vi "Begin.vi"(11 "Image Size":T1=enum."160x120") -> (0 "error out":errorcluster)   [LabVIEW 2012]
doc: "Called before other user functions, this VI is expected to open initial I/O refnums, load in file data, and do all program initialization. Notice that the <B>error out</B> terminal is simply used for data flow. Wiring it to other structures or subVIs ensures that this VI runs first."
uses:
  <vilib>/Rock Robotics/WPI/Camera/WPI_CameraImageSize.ctl
  <vilib>/Rock Robotics/WPI/DriverStation/WPI_DriverStationRobotMode2.ctl
  <vilib>/Rock Robotics/WPI/CAN/Jaguar/SubVIs/WPI_CANJaguar_ControlMode.ctl
  <vilib>/Rock Robotics/WPI/Joystick/WPI_JoystickDeviceEnum.ctl
  <vilib>/Rock Robotics/WPI/CAN/Jaguar/SubVIs/WPI_CANJaguar_SpeedReference.ctl
  Robot Global Data.vi
  <vilib>/Rock Robotics/WPI/MotorControl/WPI_MotorControlOpenCANJaguar.vi
  <vilib>/Rock Robotics/WPI/RobotDrive/WPI_RobotDriveOpen2MotorWithJaguar.vi
  <vilib>/Rock Robotics/SystemInterfaces/DIO/FPGA_DIOPWMChannel.ctl
  <vilib>/Rock Robotics/WPI/Camera/WPI_CameraWhite Balance Values.ctl
  <vilib>/Rock Robotics/WPI/Camera/WPI_CameraExposure Values.ctl
  <vilib>/Rock Robotics/WPI/Camera/WPI_CameraFrameRate.ctl
  <vilib>/Rock Robotics/WPI/SafetyOutput/WPI_SafetyOutputConfigMenu.ctl
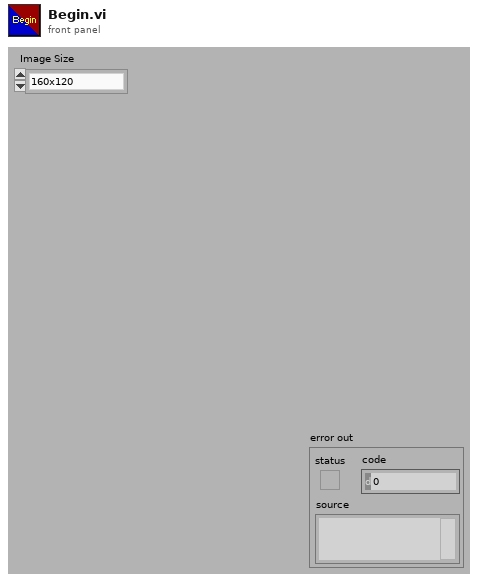
[diagram p1: front panel]
types:
  T1 = typedef "WPI_CameraImageSize.ctl" = enum16{"640x480", "320x240", "160x120"}
  T2 = typedef "WPI_CANJaguar_SpeedReference.ctl" = u8
  T3 = typedef "WPI_CANJaguar_ControlMode.ctl" = enum8{"Percent VBus", "Current", "Speed", "Position", "Voltage"}
  T4 = typedef "WPI_JoystickDeviceEnum.ctl" = enum16{"USB 1", "USB 2", "USB 3", "USB 4", "Kinect 1", "Kinect 2"}
  T5 = typedef "WPI_DriverStationRobotMode2.ctl" = enum16{"Autonomous Disabled", "Autonomous Enabled", "Teleop Disabled", "Teleop Enabled", "Timeout", "Finish", "Test Disabled", "Test Enabled"}
  T6 = typedef "WPI_CameraFrameRate.ctl" = u32
  T7 = typedef "WPI_CameraExposure Values.ctl" = enum16{"Auto", "Flicker-free 50 Hz", "Flicker-free 60 Hz", "Hold current"}
  T8 = typedef "WPI_CameraWhite Balance Values.ctl" = enum16{"Auto", "Fixed indoor", "Fixed outdoor 1", "Fixed outdoor 2", "Fixed fluorescent 1", "Fixed fluorescent 2", "Hold current"}
  T9 = typedef "WPI_CameraDevRef.ctl" = cluster{"Camera Address":string, "CameraStatus":errorcluster, "Acquire Image Notifier":refnum<notifier>}
  T10 = typedef "WPI_SafetyOutputConfigMenu.ctl" = enum16{"Enable", "Disable"}
  T11 = typedef "FPGA_DIOPWMChannel.ctl" = enum8{"PWM 1", "PWM 2", "PWM 3", "PWM 4", "PWM 5", "PWM 6", "PWM 7", "PWM 8", "PWM 9", "PWM 10", "Invalid"}
  T12 = typedef "WPI_JoystickDevRef.ctl" = cluster{"Device":T4}
  T13 = typedef "WPI_RobotDriveDevRef.ctl" = cluster{"DevStatus":errorcluster, "Motors[]":T14[], "Square Inputs":bool, "Max Output":dbl, "Isochronous":bool}
  T14 = typedef "WPI_MotorControlDeviceRef.ctl" = cluster{"DeviceStatus":errorcluster, "Type":enum16{"PWM", "CAN"}, "PWM":cluster{"Digital Module":T15, "PWM Channel":T11, "DeadBand":T16}, "CAN":cluster{"Device Number":u8, "Control Mode":T3, "Semaphore":T17, "Max Vout":dbl}, "Invert":bool, "TransformRef":T18, "InvTransformRef":T18}
  T15 = typedef "FPGA_TypedefDigitalModule.ctl" = enum16{"Digital Module 1", "Digital Module 2"}
  T16 = typedef "WPI_PWMDeadband.ctl" = cluster{"Name":string, "maxPositivePwm":i32, "minPositivePwm":i32, "centerPwm":i32, "maxNegativePwm":i32, "minNegativePwm":i32, "angularRange":u16}
  T17 = typedef "Semaphore RefNum" = refnum<k1>
  T18 = typedef "WPI_PWMTransform_ConPane.ctl" = refnum<vi>
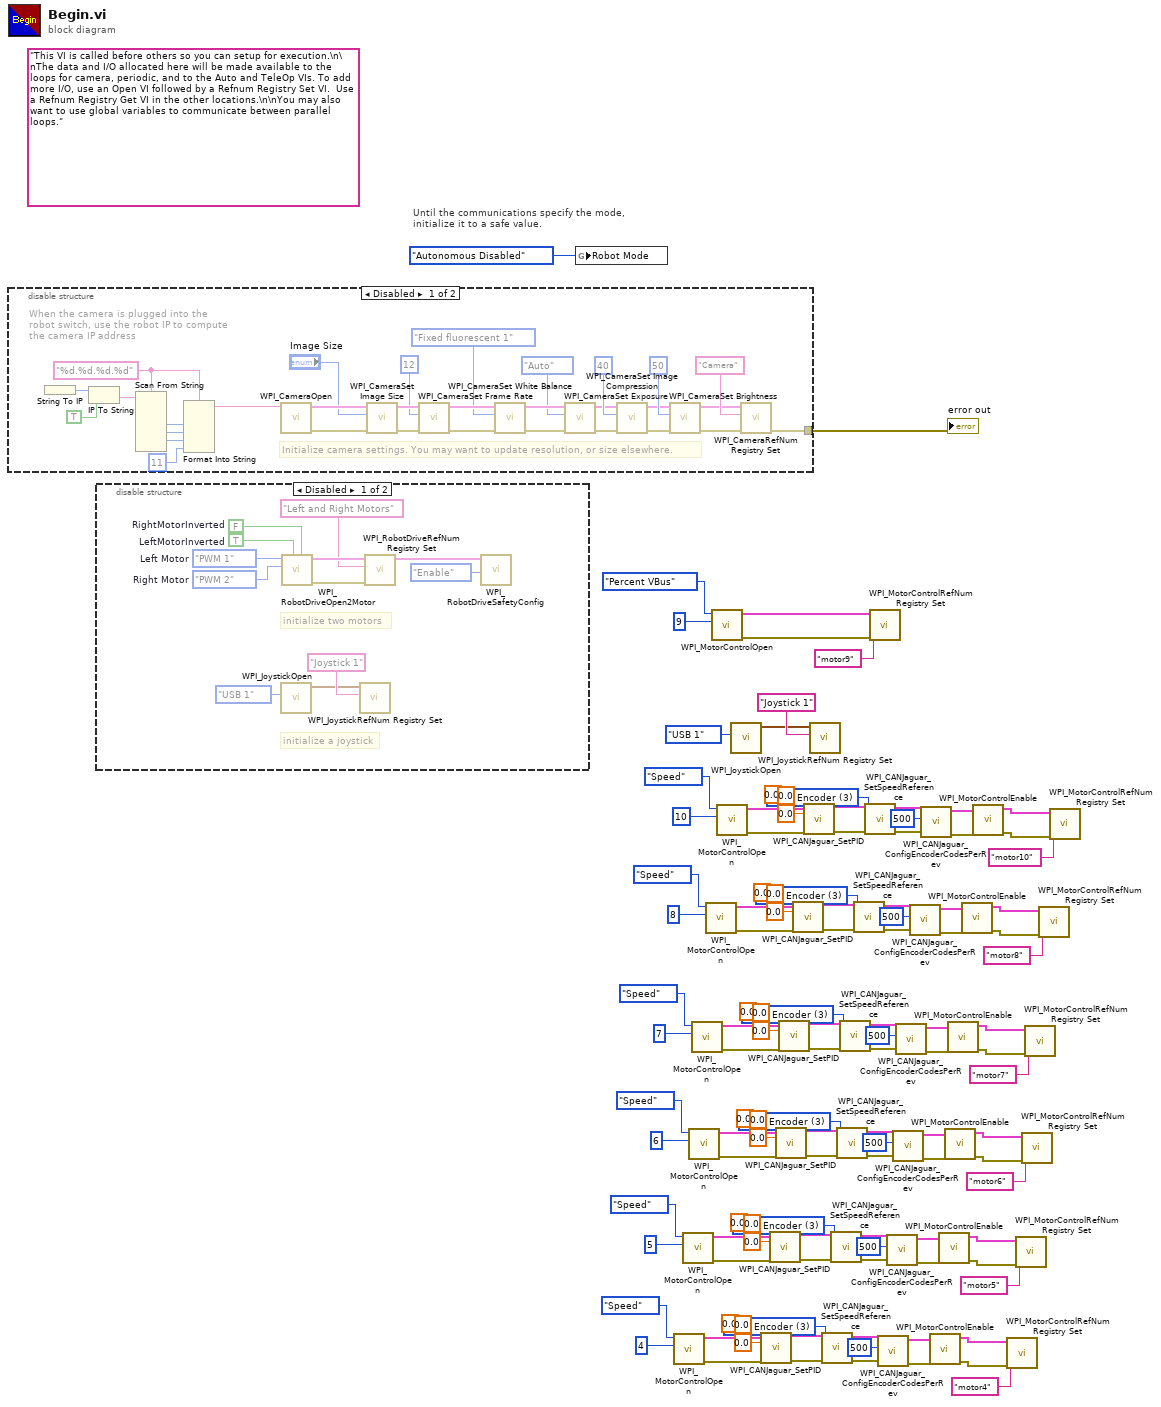
[diagram p0: block diagram]
diagram:
  w9 = T2 3 items=["Encoder"=0, "Inv Encoder"=2, "Quad Encoder"=3, "None"=255] ("Speed Reference")
  w27 = T2 3 items=["Encoder"=0, "Inv Encoder"=2, "Quad Encoder"=3, "None"=255] ("Speed Reference")
  w45 = T2 3 items=["Encoder"=0, "Inv Encoder"=2, "Quad Encoder"=3, "None"=255] ("Speed Reference")
  w63 = T2 3 items=["Encoder"=0, "Inv Encoder"=2, "Quad Encoder"=3, "None"=255] ("Speed Reference")
  w81 = T2 3 items=["Encoder"=0, "Inv Encoder"=2, "Quad Encoder"=3, "None"=255] ("Speed Reference")
  w99 = T2 3 items=["Encoder"=0, "Inv Encoder"=2, "Quad Encoder"=3, "None"=255] ("Speed Reference")
  (unwired) "This VI is called before others so you can setup for execution.\n\nThe data and I/O allocated here will be made available to the loops for camera, periodic, and to the Auto and TeleOp VIs. To add more I/O, use an Open VI followed by a Refnum Registry Set VI.  Use a Refnum Registry Get VI in the other locations.\n\nYou may also want to use global variables to communicate between parallel loops."
  # "Until the communications specify the mode,\ninitialize it to a safe value."
  n1 = disable-structure shown="Disabled" {
    disable-tunnel: [w119 _] -> w117
    frame Disabled {
      w121 = "%d.%d.%d.%d" ("format string")
      # "When the camera is plugged into the\nrobot switch, use the robot IP to compute\nthe camera IP address"
      # "Initialize camera settings. You may want to update resolution, or size elsewhere."
      n2 = String To IP() -> (0:w128:u32)  [unwired: 1 in]
      n3 = IP To String(1:TRUE ("dot notation? (F)"), 2:w128) -> (0:w126:string)
      n4 = Scan From String(format string=w121, input string=w126) -> (output 1=w125:i32, output 2=w124:i32, output 3=w123:i32)  [unwired: 7 in, 3 out]
      n5 = Format Into String(format string=w121, w125, w124, w123, 11 ("Compression")) -> (resulting string=w120:string)  [unwired: 2 in, 1 out]
      n6 = call <vilib>:"WPI_CameraOpen.vi"("Camera Address"=w120) -> ("error out"=w140:errorcluster, "CameraDevRef"=w141:T9)  [unwired: 1 in, 8 out]
      n7 = call <vilib>:"WPI_CameraSet Image Size.vi"("error in (no error)"=w140, "Image Size"="Image Size", "CameraDevRef"=w141) -> ("error out"=w139:errorcluster, "CameraDevRef Out"=w142:T9)  [unwired: 7 out]
      n8 = call <vilib>:"WPI_CameraSet Frame Rate.vi"("error in (no error)"=w139, "Frame Rate (fps)"=T6 12, "CameraDevRef"=w142) -> ("error out"=w138:errorcluster, "CameraDevRef Out"=w144:T9)  [unwired: 7 out]
      n9 = call <vilib>:"WPI_CameraSet White Balance.vi"("error in (no error)"=w138, "White Balance"=WPI_CameraWhite_Balance_Values."Fixed fluorescent 1", "CameraDevRef"=w144) -> ("error out"=w137:errorcluster, "CameraDevRef Out"=w143:T9)  [unwired: 7 out]
      n10 = call <vilib>:"WPI_CameraSet Exposure.vi"("error in (no error)"=w137, "Exposure"=WPI_CameraExposure_Values."Auto", "CameraDevRef"=w143) -> ("error out"=w136:errorcluster, "CameraDevRef Out"=w146:T9)  [unwired: 7 out]
      n11 = call <vilib>:"WPI_CameraSet Image Compression.vi"("error in (no error)"=w136, "Compression"=40, "CameraDevRef"=w146) -> ("error out"=w135:errorcluster, "CameraDevRef Out"=w145:T9)  [unwired: 7 out]
      n12 = call <vilib>:"WPI_CameraSet Brightness.vi"("error in (no error)"=w135, "Brightness"=50, "CameraDevRef"=w145) -> ("error out"=w133:errorcluster, "CameraDevRef Out"=w134:T9)  [unwired: 7 out]
      n13 = call <vilib>:"WPI_CameraRefNum Registry Set.vi"("error in (no error)"=w133, "refnum name"="Camera", "CameraDevRef"=w134) -> ("error out"=w119:errorcluster)  [unwired: 8 out]
    }
    frame Enabled {
    }
  }
  "error out" <- w117
  n14 = disable-structure shown="Disabled" {
    frame Disabled {
      w155 = FPGA_DIOPWMChannel."PWM 2"  # Right Motor
      w156 = FPGA_DIOPWMChannel."PWM 1"  # Left Motor
      w160 = TRUE  # LeftMotorInverted
      w161 = FALSE  # RightMotorInverted
      # "initialize a joystick"
      # "initialize two motors"
      n15 = call <vilib>:"WPI_JoystickOpen.vi"("JoystickDevice"=WPI_JoystickDeviceEnum."USB 1") -> ("JoystickDevRef"=w151:T12)  [unwired: 10 in]
      n16 = call-poly <vilib>:"WPI_RobotDriveOpen2Motor.vi"("Right Motor Inverted"=w161, "Left Motor Inverted"=w160, "Right Motor"=w155, "Left Motor"=w156) -> ("error out"=w157:errorcluster, "RobotDriveDevRef"=w159:T13)  [unwired: 1 in, 5 out]
      n17 = call <vilib>:"WPI_JoystickRefNum Registry Set.vi"("refnum name"="Joystick 1", "JoystickDevRef"=w151) -> ()  [unwired: 8 in, 2 out]
      n18 = call <vilib>:"WPI_RobotDriveRefNum Registry Set.vi"("error in (no error)"=w157, "refnum name"="Left and Right Motors", "RobotDriveDevRef"=w159) -> ("RobotDriveDevRef"=w154:T13)  [unwired: 8 out]
      n19 = call <vilib>:"WPI_RobotDriveSafetyConfig.vi"("mode"=WPI_SafetyOutputConfigMenu."Enable", "RobotDriveDevRef"=w154) -> ()  [unwired: 8 in, 2 out]
    }
    frame Enabled {
    }
  }
  n20 = global write "Robot Global Data.vi" "Robot Mode"(WPI_DriverStationRobotMode2."Autonomous Disabled" ("Robot Mode")) -> ()
  n21 = call-poly <vilib>:"WPI_MotorControlOpen.vi"("Device Number"=u8 4, "Control Mode"=WPI_CANJaguar_ControlMode."Speed") -> ("error out"=w15:errorcluster, "MotorControlDeviceRef"=w16:T14)  [unwired: 8 in]
  n22 = call-poly <vilib>:"WPI_MotorControlOpen.vi"("Device Number"=u8 5, "Control Mode"=WPI_CANJaguar_ControlMode."Speed") -> ("error out"=w33:errorcluster, "MotorControlDeviceRef"=w34:T14)  [unwired: 8 in]
  n23 = call-poly <vilib>:"WPI_MotorControlOpen.vi"("Device Number"=u8 6, "Control Mode"=WPI_CANJaguar_ControlMode."Speed") -> ("error out"=w51:errorcluster, "MotorControlDeviceRef"=w52:T14)  [unwired: 8 in]
  n24 = call-poly <vilib>:"WPI_MotorControlOpen.vi"("Device Number"=u8 7, "Control Mode"=WPI_CANJaguar_ControlMode."Speed") -> ("error out"=w69:errorcluster, "MotorControlDeviceRef"=w70:T14)  [unwired: 8 in]
  n25 = call-poly <vilib>:"WPI_MotorControlOpen.vi"("Device Number"=u8 8, "Control Mode"=WPI_CANJaguar_ControlMode."Speed") -> ("error out"=w87:errorcluster, "MotorControlDeviceRef"=w88:T14)  [unwired: 8 in]
  n26 = call-poly <vilib>:"WPI_MotorControlOpen.vi"("Device Number"=u8 9, "Control Mode"=WPI_CANJaguar_ControlMode."Percent VBus") -> ("error out"=w113:errorcluster, "MotorControlDeviceRef"=w114:T14)  [unwired: 8 in]
  n27 = call-poly <vilib>:"WPI_MotorControlOpen.vi"("Device Number"=u8 10, "Control Mode"=WPI_CANJaguar_ControlMode."Speed") -> ("error out"=w105:errorcluster, "MotorControlDeviceRef"=w106:T14)  [unwired: 8 in]
  n28 = call <vilib>:"WPI_JoystickOpen.vi"("JoystickDevice"=WPI_JoystickDeviceEnum."USB 1") -> ("JoystickDevRef"=w110:T12)  [unwired: 10 in]
  n29 = call <vilib>:"WPI_CANJaguar_SetPID.vi"("CAN Jaguar Ref"=w16, "P"=0.0, "I"=0.0, "D"=0.0, "error in (no error)"=w15) -> ("CAN Jaguar Ref Out"=w11:T14, "error out"=w10:errorcluster)  [unwired: 9 in]
  n30 = call <vilib>:"WPI_CANJaguar_SetPID.vi"("CAN Jaguar Ref"=w34, "P"=0.0, "I"=0.0, "D"=0.0, "error in (no error)"=w33) -> ("CAN Jaguar Ref Out"=w29:T14, "error out"=w28:errorcluster)  [unwired: 9 in]
  n31 = call <vilib>:"WPI_CANJaguar_SetPID.vi"("CAN Jaguar Ref"=w52, "P"=0.0, "I"=0.0, "D"=0.0, "error in (no error)"=w51) -> ("CAN Jaguar Ref Out"=w47:T14, "error out"=w46:errorcluster)  [unwired: 9 in]
  n32 = call <vilib>:"WPI_CANJaguar_SetPID.vi"("CAN Jaguar Ref"=w70, "P"=0.0, "I"=0.0, "D"=0.0, "error in (no error)"=w69) -> ("CAN Jaguar Ref Out"=w65:T14, "error out"=w64:errorcluster)  [unwired: 9 in]
  n33 = call <vilib>:"WPI_CANJaguar_SetPID.vi"("CAN Jaguar Ref"=w88, "P"=0.0, "I"=0.0, "D"=0.0, "error in (no error)"=w87) -> ("CAN Jaguar Ref Out"=w83:T14, "error out"=w82:errorcluster)  [unwired: 9 in]
  n34 = call <vilib>:"WPI_CANJaguar_SetPID.vi"("CAN Jaguar Ref"=w106, "P"=0.0, "I"=0.0, "D"=0.0, "error in (no error)"=w105) -> ("CAN Jaguar Ref Out"=w101:T14, "error out"=w100:errorcluster)  [unwired: 9 in]
  n35 = call <vilib>:"WPI_JoystickRefNum Registry Set.vi"("refnum name"="Joystick 1", "JoystickDevRef"=w110) -> ()  [unwired: 8 in, 2 out]
  n36 = call <vilib>:"WPI_CANJaguar_SetSpeedReference.vi"("error in (no error)"=w10, "Speed Reference"=w9, "CAN Jaguar Ref"=w11) -> ("error out"=w7:errorcluster, "CAN Jaguar Ref Out"=w8:T14)  [unwired: 7 in]
  n37 = call <vilib>:"WPI_CANJaguar_SetSpeedReference.vi"("error in (no error)"=w28, "Speed Reference"=w27, "CAN Jaguar Ref"=w29) -> ("error out"=w25:errorcluster, "CAN Jaguar Ref Out"=w26:T14)  [unwired: 7 in]
  n38 = call <vilib>:"WPI_CANJaguar_SetSpeedReference.vi"("error in (no error)"=w46, "Speed Reference"=w45, "CAN Jaguar Ref"=w47) -> ("error out"=w43:errorcluster, "CAN Jaguar Ref Out"=w44:T14)  [unwired: 7 in]
  n39 = call <vilib>:"WPI_CANJaguar_SetSpeedReference.vi"("error in (no error)"=w64, "Speed Reference"=w63, "CAN Jaguar Ref"=w65) -> ("error out"=w61:errorcluster, "CAN Jaguar Ref Out"=w62:T14)  [unwired: 7 in]
  n40 = call <vilib>:"WPI_CANJaguar_SetSpeedReference.vi"("error in (no error)"=w82, "Speed Reference"=w81, "CAN Jaguar Ref"=w83) -> ("error out"=w79:errorcluster, "CAN Jaguar Ref Out"=w80:T14)  [unwired: 7 in]
  n41 = call <vilib>:"WPI_CANJaguar_SetSpeedReference.vi"("error in (no error)"=w100, "Speed Reference"=w99, "CAN Jaguar Ref"=w101) -> ("error out"=w97:errorcluster, "CAN Jaguar Ref Out"=w98:T14)  [unwired: 7 in]
  n42 = call <vilib>:"WPI_MotorControlRefNum Registry Set.vi"("error in (no error)"=w113, "refnum name"="motor9", "MotorControlDevRef"=w114) -> ()  [unwired: 7 in, 2 out]
  n43 = call <vilib>:"WPI_CANJaguar_ConfigEncoderCodesPerRev.vi"("error in (no error)"=w7, "Encoder Codes Per Rev"=u16 500, "CAN Jaguar Ref"=w8) -> ("error out"=w5:errorcluster, "CAN Jaguar Ref Out"=w4:T14)  [unwired: 7 in]
  n44 = call <vilib>:"WPI_CANJaguar_ConfigEncoderCodesPerRev.vi"("error in (no error)"=w25, "Encoder Codes Per Rev"=u16 500, "CAN Jaguar Ref"=w26) -> ("error out"=w23:errorcluster, "CAN Jaguar Ref Out"=w22:T14)  [unwired: 7 in]
  n45 = call <vilib>:"WPI_CANJaguar_ConfigEncoderCodesPerRev.vi"("error in (no error)"=w43, "Encoder Codes Per Rev"=u16 500, "CAN Jaguar Ref"=w44) -> ("error out"=w41:errorcluster, "CAN Jaguar Ref Out"=w40:T14)  [unwired: 7 in]
  n46 = call <vilib>:"WPI_CANJaguar_ConfigEncoderCodesPerRev.vi"("error in (no error)"=w61, "Encoder Codes Per Rev"=u16 500, "CAN Jaguar Ref"=w62) -> ("error out"=w59:errorcluster, "CAN Jaguar Ref Out"=w58:T14)  [unwired: 7 in]
  n47 = call <vilib>:"WPI_CANJaguar_ConfigEncoderCodesPerRev.vi"("error in (no error)"=w79, "Encoder Codes Per Rev"=u16 500, "CAN Jaguar Ref"=w80) -> ("error out"=w77:errorcluster, "CAN Jaguar Ref Out"=w76:T14)  [unwired: 7 in]
  n48 = call <vilib>:"WPI_CANJaguar_ConfigEncoderCodesPerRev.vi"("error in (no error)"=w97, "Encoder Codes Per Rev"=u16 500, "CAN Jaguar Ref"=w98) -> ("error out"=w95:errorcluster, "CAN Jaguar Ref Out"=w94:T14)  [unwired: 7 in]
  n49 = call <vilib>:"WPI_MotorControlEnable.vi"("error in (no error)"=w5, "CAN Jaguar Ref"=w4) -> ("error out"=w2:errorcluster, "CAN Jaguar Ref Out"=w3:T14)  [unwired: 8 in]
  n50 = call <vilib>:"WPI_MotorControlEnable.vi"("error in (no error)"=w23, "CAN Jaguar Ref"=w22) -> ("error out"=w20:errorcluster, "CAN Jaguar Ref Out"=w21:T14)  [unwired: 8 in]
  n51 = call <vilib>:"WPI_MotorControlEnable.vi"("error in (no error)"=w41, "CAN Jaguar Ref"=w40) -> ("error out"=w38:errorcluster, "CAN Jaguar Ref Out"=w39:T14)  [unwired: 8 in]
  n52 = call <vilib>:"WPI_MotorControlEnable.vi"("error in (no error)"=w59, "CAN Jaguar Ref"=w58) -> ("error out"=w56:errorcluster, "CAN Jaguar Ref Out"=w57:T14)  [unwired: 8 in]
  n53 = call <vilib>:"WPI_MotorControlEnable.vi"("error in (no error)"=w77, "CAN Jaguar Ref"=w76) -> ("error out"=w74:errorcluster, "CAN Jaguar Ref Out"=w75:T14)  [unwired: 8 in]
  n54 = call <vilib>:"WPI_MotorControlEnable.vi"("error in (no error)"=w95, "CAN Jaguar Ref"=w94) -> ("error out"=w92:errorcluster, "CAN Jaguar Ref Out"=w93:T14)  [unwired: 8 in]
  n55 = call <vilib>:"WPI_MotorControlRefNum Registry Set.vi"("error in (no error)"=w2, "refnum name"="motor4", "MotorControlDevRef"=w3) -> ()  [unwired: 7 in, 2 out]
  n56 = call <vilib>:"WPI_MotorControlRefNum Registry Set.vi"("error in (no error)"=w20, "refnum name"="motor5", "MotorControlDevRef"=w21) -> ()  [unwired: 7 in, 2 out]
  n57 = call <vilib>:"WPI_MotorControlRefNum Registry Set.vi"("error in (no error)"=w38, "refnum name"="motor6", "MotorControlDevRef"=w39) -> ()  [unwired: 7 in, 2 out]
  n58 = call <vilib>:"WPI_MotorControlRefNum Registry Set.vi"("error in (no error)"=w56, "refnum name"="motor7", "MotorControlDevRef"=w57) -> ()  [unwired: 7 in, 2 out]
  n59 = call <vilib>:"WPI_MotorControlRefNum Registry Set.vi"("error in (no error)"=w74, "refnum name"="motor8", "MotorControlDevRef"=w75) -> ()  [unwired: 7 in, 2 out]
  n60 = call <vilib>:"WPI_MotorControlRefNum Registry Set.vi"("error in (no error)"=w92, "refnum name"="motor10", "MotorControlDevRef"=w93) -> ()  [unwired: 7 in, 2 out]
